vi "Global 1.vi"() -> ()   [LabVIEW 2009]
uses:
  spotfindersettings.ctl
  Settings.ctl
panel:
  out "StandardSettings":T1={"threshold"={"max"=0, "min"=0}, "RGB or false color"=TRUE, "16bit"=TRUE, "log/lin axis"=0, "spotsize button"=TRUE, "Pixelsize"=10, "autoscale x"=TRUE, "autoscale y"=TRUE, "correlation"=TRUE, "ADC-Resolution"=128, "F2-lifetime"={"display tau"=FALSE, "display F2"=FALSE, "Palette Number lifetime"=enum."Temperature", "Palette Number F2"=enum."Rainbow", "max tau-Value"=10.0, "min tau-Value"=0.0, "max F2-Value"=1.0, "min F2-Value"=0.0}, "TAC-Window 1"=60, "TAC-Window 2"=0, "false color palette"={"1"=0, "2"=0, "3"=0, "4"=0, "5"=0, "6"=0, "7"=0, "8"=0, "8 2"=0, "8 3"=0, "8 4"=0, "8 5"=0}} {"false color palette"."8 5" format="%.0x"; "false color palette"."8 4" format="%.0x"; "false color palette"."8 3" format="%.0x"; "false color palette"."8 2" format="%.0x"; "false color palette"."8" format="%.0x"; "false color palette"."7" format="%.0x"; "false color palette"."6" format="%.0x"; "false color palette"."5" format="%.0x"; "false color palette"."4" format="%.0x"; "false color palette"."3" format="%.0x"; "false color palette"."2" format="%.0x"; "false color palette"."1" format="%.0x"; "log/lin axis" items=["linear y-axis", "log y-axis"]; "F2-lifetime"."min tau-Value" format="%.2f"; "F2-lifetime"."max tau-Value" format="%.2f"; "F2-lifetime"."max F2-Value" format="%.2f"; "F2-lifetime"."min F2-Value" format="%.2f"}
  out "spotfinding settings":T2={"show all"=FALSE, "threshold/morph"=FALSE, "particle filter"=FALSE, "spot marks"=FALSE, "close filter"=FALSE, "connectivity 4/8"=FALSE, "range"={"Lower value"=30.0, "Upper value"=30.0}, "PSF-size"=0, "Parameters"=[]} {"range"."Upper value" format="%.2f"; "range"."Lower value" format="%.2f"; "Parameters"."Upper Value" format="%.2f"; "Parameters"."Lower Value" format="%.2f"}
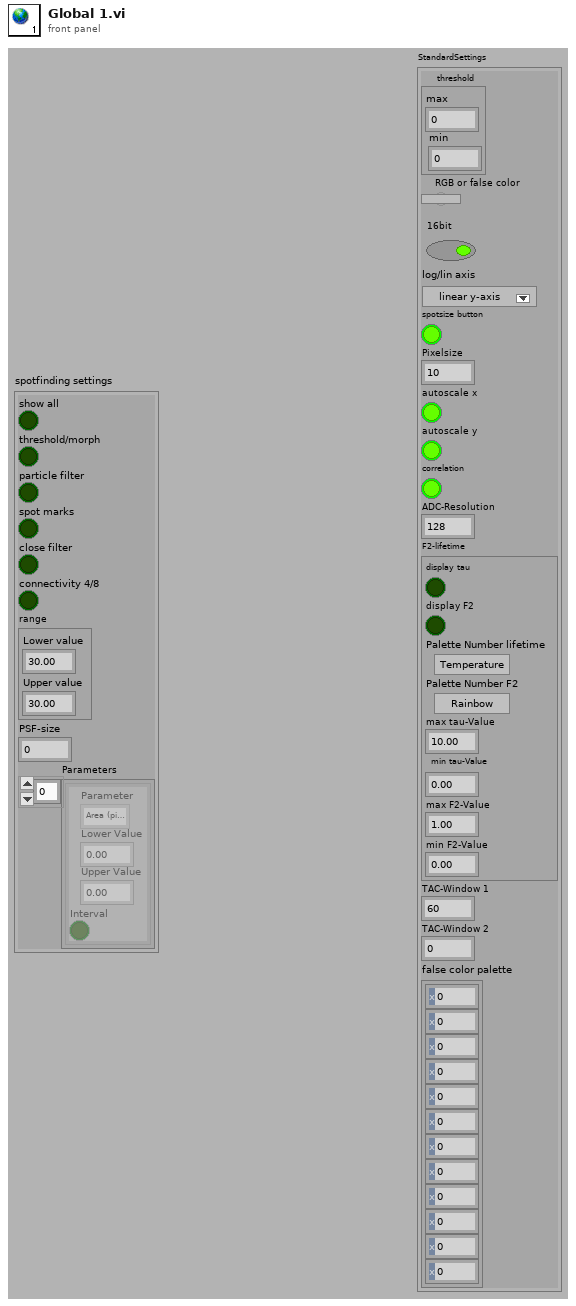
[diagram p1: front panel]
types:
  T1 = typedef "Settings.ctl" = cluster{"threshold":cluster{"max":u32, "min":u32}, "RGB or false color":bool, "16bit":bool, "log/lin axis":u16, "spotsize button":bool, "Pixelsize":u16, "autoscale x":bool, "autoscale y":bool, "correlation":bool, "ADC-Resolution":i32, "F2-lifetime":cluster{"display tau":bool, "display F2":bool, "Palette Number lifetime":enum32{"Gray", "Binary", "Gradient", "Rainbow", "Temperature"}, "Palette Number F2":enum32{"Gray", "Binary", "Gradient", "Rainbow", "Temperature"}, "max tau-Value":dbl, "min tau-Value":dbl, "max F2-Value":dbl, "min F2-Value":dbl}, "TAC-Window 1":u16, "TAC-Window 2":u16, "false color palette":cluster{"1":u32, "2":u32, "3":u32, "4":u32, "5":u32, "6":u32, "7":u32, "8":u32, "8 2":u32, "8 3":u32, "8 4":u32, "8 5":u32}}
  T2 = typedef "spotfindersettings.ctl" = cluster{"show all":bool, "threshold/morph":bool, "particle filter":bool, "spot marks":bool, "close filter":bool, "connectivity 4/8":bool, "range":cluster{"Lower value":sgl, "Upper value":sgl}, "PSF-size":i32, "Parameters":cluster{"Parameter":enum32{"Area (pixels)", "Area (calibrated)", "Number of holes", "Holes area (pixels)", "Total area (pixels)", "Scanned area (pixels)", "Ratio Area/Scanned area (%)", "Ratio Area/Total area (%)", "Center of mass (X)", "Center of mass (Y)", "Left column (X)", "Upper row (Y)", "Right column (X)", "Lower row (Y)", "Width (pixels)", "Height (pixels)", "Longest segment length", "Longest segment left column (X)", "Longest segment top row  (Y)", "Perimeter", "Holes perimeter", "SumX", "SumY", "SumXX", "SumYY", "SumXY", "Corrected projection X", "Corrected projection Y", "Moment of inertia Ixx", "Moment of inertia Iyy", "Moment of inertia Ixy", "Mean chord X", "Mean chord Y", "Max intercept", "Mean intercept perpendicular", "Particle orientation", "Equivalent ellipse minor axis", "Ellipse major axis", "Ellipse minor axis", "Ratio of equivalent ellipse axis", "Rectangle big side", "Rectangle small side", "Ratio of equivalent rectangle sides", "Elongation factor", "Compactness factor", "Heywood circularity factor", "Type factor", "Hydraulic radius", "Waddel disk diameter", "Diagonal"}, "Lower Value":sgl, "Upper Value":sgl, "Interval":bool}[]}
diagram:
